vi "Read_Single_Reg.vi"(2 "Read I2C Address":u8 format="%x", 3 "USB DAQ Address":i32 format="%x", 4 "Reg No":u8 format="%x") -> (0 "Status String":string="ERROR COMMUNICATING WITH DEVICE", 1 "Read Result":u16)   [LabVIEW 2011]
doc: "This VI is used to read a single register. Device address, I2C device address, and register number are converted and concatenated into a single mnemonic command string, which is input to the \"RunMnemCmd\" VI. The VI outputs the results of the read and also performs error-checks on the ACKS array. If an error is found, the VI reports to Main and displays an error message."
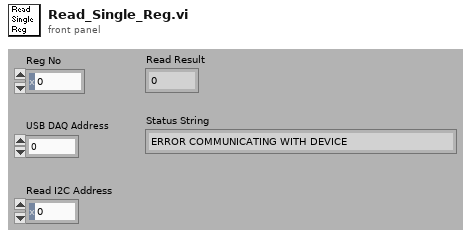
[diagram p1: front panel]
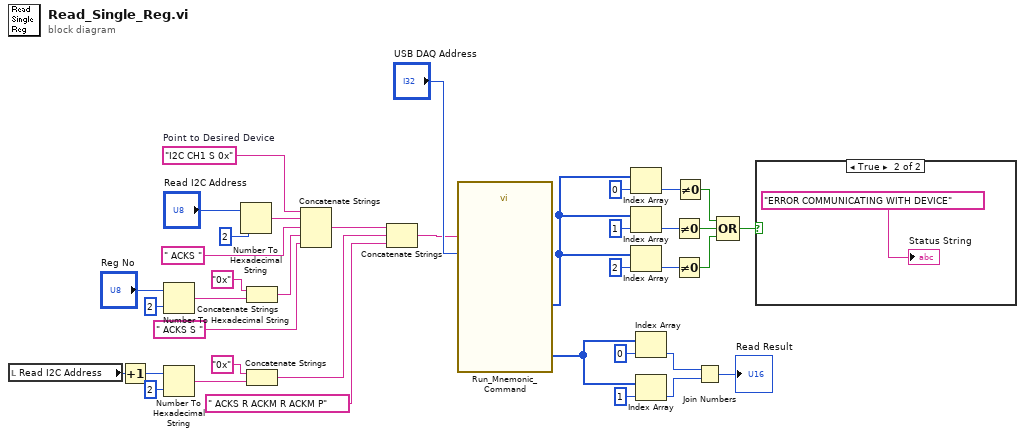
[diagram p0: block diagram]
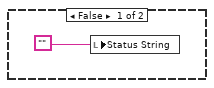
[diagram p2: hidden frame]
diagram:
  w30 = "I2C CH1 S 0x"  # Point to Desired Device
  n1 = local read "Read I2C Address"() -> (w12:u8)
  n2 = Increment(x=w12) -> (x+1=w21:u8)
  n3 = Number To Hexadecimal String(1:i16 2 ("width (-)"), 2:"Reg No") -> (0:w25:string)
  n4 = Number To Hexadecimal String(1:i16 2 ("width (-)"), 2:w21) -> (0:w15:string)
  n5 = Number To Hexadecimal String(1:i16 2 ("width (-)"), 2:"Read I2C Address") -> (0:w29:string)
  n6 = Concatenate Strings("0x" ("string"), w25) -> (w24:string)
  n7 = Concatenate Strings("0x" ("string"), w15) -> (w14:string)
  n8 = Concatenate Strings(w30, w29, " ACKS " ("string"), w24, " ACKS S " ("string")) -> (w22:string)
  n9 = Concatenate Strings(w22, w14, " ACKS R ACKM R ACKM P" ("string")) -> (w19:string)
  n10 = call "Run_Mnemonic_Command.vi"("command string"=w19, "Device address"="USB DAQ Address") -> ("ACKS-array"=w8:u8[], "result-array"=w33:u8[])  [unwired: 2 in, 3 out]
  n11 = Index Array(array=w8, index=0) -> (element=w7:u8)
  n12 = Index Array(array=w8, index=1) -> (element=w2:u8)
  n13 = Index Array(array=w8, index=2) -> (element=w5:u8)
  n14 = Index Array(array=w33, index=0) -> (element=w35:u8)
  n15 = Index Array(array=w33, index=1) -> (element=w34:u8)
  n16 = Not Equal To 0?(x=w2) -> (x != 0?=w6:bool)
  n17 = Not Equal To 0?(x=w5) -> (x != 0?=w4:bool)
  n18 = Not Equal To 0?(x=w7) -> (x != 0?=w3:bool)
  n19 = Join Numbers(hi=w35, lo=w34) -> ((hi.lo)=→"Read Result":u16)
  n20 = Compound Arithmetic op=OR(w3, w6, w4) -> (w1:bool)
  n21 = case shown="True" w1 {
    frame False {
      n22 = local write "Status String"("") -> ()
    }
    frame True {
      "Status String" <- "ERROR COMMUNICATING WITH DEVICE"
    }
  }
